vi "Encapsulation to LEIN.vi"(7 "Data and header":u8[](array[numeric]), 11 "error in (no error)":errorcluster) -> (6 "LEIN OK":bool, 8 "CMD out":T1={"SID"=0, "ANF"=FALSE, "CMD"=enum."TASK", "DATA"=[]}, 14 "Data Length":u32, 15 "error out":errorcluster)   [LabVIEW 2011]
uses:
  Defenitions/LEIN CMD Cluster.ctl
  Defenitions/LEIN CMD List.ctl
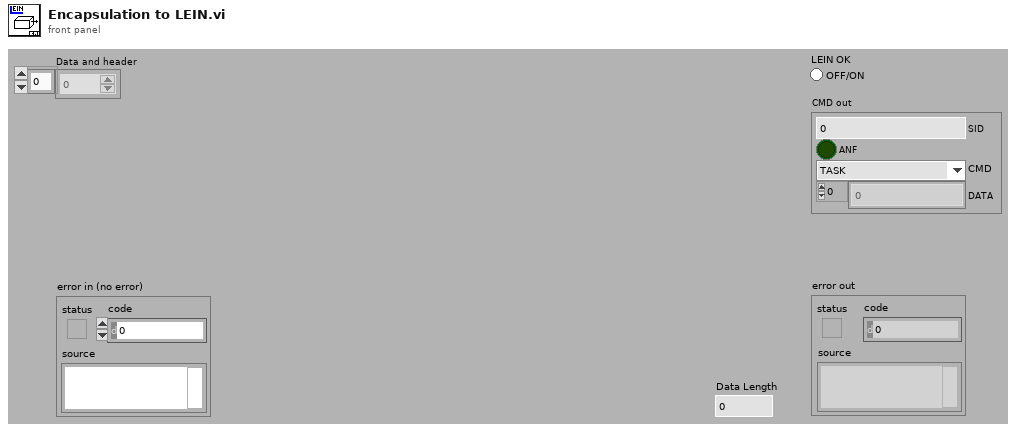
[diagram p1: front panel]
types:
  T1 = typedef "LEIN CMD Cluster.ctl" = cluster{"SID":u8, "ANF":bool, "CMD":T2, "DATA":u8[]}
  T2 = typedef "LEIN CMD List.ctl" = enum8{"ACTI", "TASK", "RES0", "STAT", "RES1", "RES2", "RES3", "USER"}
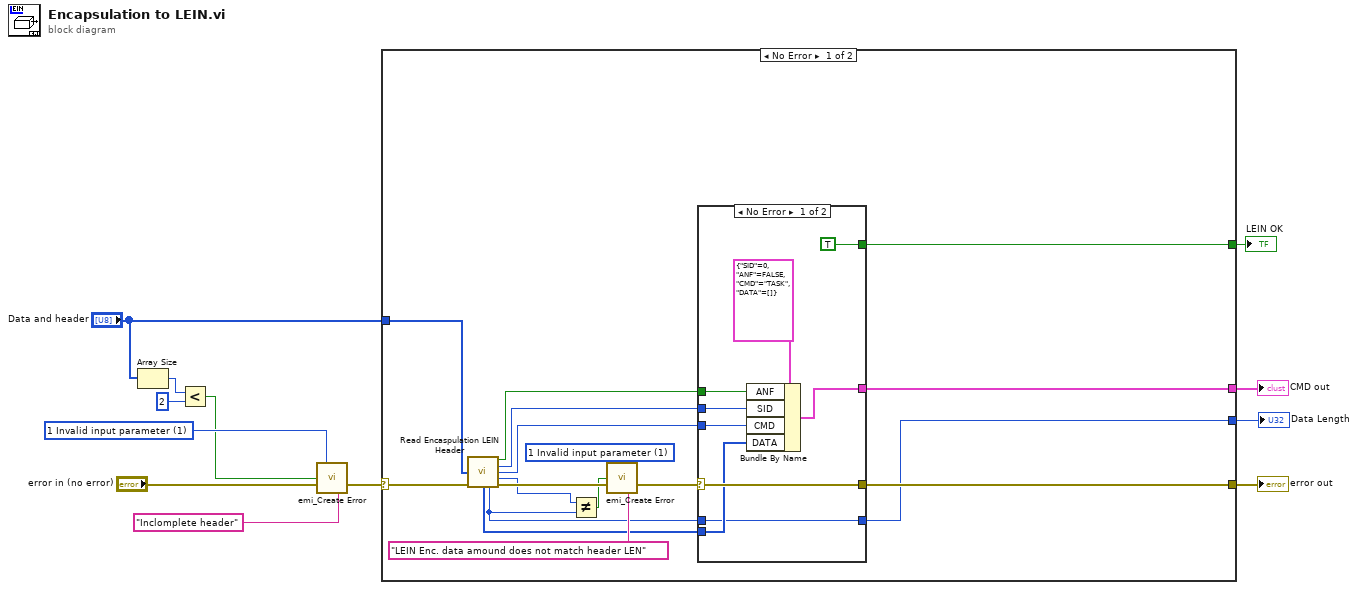
[diagram p0: block diagram]
diagram:
  w11 = 1 items=["0 No Error"=0, "1 Invalid input parameter"=1, "6 Generic file IO "=6, "7 File not Found"=7, "35 Generic Pring Error"=35, "37 Device not Found"=37, "39 Device Unit Error"=39, "40 Could fot Open Device"=40, "42 Generic Error"=42, "52 Unknown Message"=52, "98 Bad File type"=98, "99 Bad File Version"=99, "100 Bad Data in File"=100, "1018 Unspecefied Error"=1018, "1041 Incorrect Password"=1041, "1043 Feature not in this version"=1043, "1109 Unsuported Data type"=1109, "1444 Did not close sucessfully"=1444] ("Error Code")
  n1 = Array Size(array="Data and header") -> (size(s)=w5:i32)
  n2 = Less?(x=w5, y=2) -> (x < y?=w8:bool)
  n3 = call "emi_Create Error.vi"("Error Code"=w11, "Error(T)"=w8, "error in (no error)"="error in (no error)", "Append String(\"\")"="Inclomplete header" ("Append String(\"\")")) -> ("error out"=w7:errorcluster)  [unwired: 11 in]
  n4 = case shown="No Error" w7 {
    selector: w7 -> [w29 w40]
    tunnel: [w19 w40] -> w6
    tunnel: "Data and header" -> [w28 _]
    tunnel: [w16 _] -> w3
    tunnel: [w15 _] -> w2
    tunnel: [w14 _] -> w1
    frame No Error {
      w22 = 1 items=["0 No Error"=0, "1 Invalid input parameter"=1, "6 Generic file IO "=6, "7 File not Found"=7, "35 Generic Pring Error"=35, "37 Device not Found"=37, "39 Device Unit Error"=39, "40 Could fot Open Device"=40, "42 Generic Error"=42, "52 Unknown Message"=52, "98 Bad File type"=98, "99 Bad File Version"=99, "100 Bad Data in File"=100, "1018 Unspecefied Error"=1018, "1041 Incorrect Password"=1041, "1043 Feature not in this version"=1043, "1109 Unsuported Data type"=1109, "1444 Did not close sucessfully"=1444] ("Error Code")
      n5 = call "Read Encaspulation LEIN Header.vi"("LEIN encapsulated Data and header"=w28, "error in (no error)"=w29) -> ("ACK"=w27:bool, "SID"=w26:u8, "CMD"=w25:u8, "LEN"=w13:u8, "Data"=w18:u8[], "Data len"=w17:i32, "error out"=w24:errorcluster)  [unwired: 7 in]
      n6 = Not Equal?(x=w13, y=w17) -> (x != y?=w23:bool)
      n7 = call "emi_Create Error.vi"("Error Code"=w22, "Error(T)"=w23, "error in (no error)"=w24, "Append String(\"\")"="LEIN Enc. data amound does not match header LEN" ("Append String(\"\")")) -> ("error out"=w20:errorcluster)  [unwired: 11 in]
      n8 = case shown="No Error" w20 {
        selector: w20 -> [w35 w39]
        tunnel: w27 -> [w38 _]
        tunnel: w26 -> [w37 _]
        tunnel: w25 -> [w36 _]
        tunnel: [w35 w39] -> w19
        tunnel: w18 -> [w34 _]
        tunnel: w17 -> [w33 _]
        tunnel: [w33 _] -> w15
        tunnel: [w32 _] -> w16
        tunnel: [TRUE _] -> w14
        frame No Error {
          n9 = Bundle By Name(cluster=T1 {"SID"=0, "ANF"=FALSE, "CMD"=enum."TASK", "DATA"=[]} ("CMD out"), "ANF"=w38, "SID"=w37, "CMD"=w36, "DATA"=w34) -> (w32:T1)
        }
        frame Error {
        }
      }
    }
    frame Error {
    }
  }
  "CMD out" <- w3
  "error out" <- w6
  "Data Length" <- w2
  "LEIN OK" <- w1
